vi "SetSheetColor.vi"() -> ()   [LabVIEW 2014]
panel:
  out "A0 2":string[][](table)
  in  "活动单元格:单元格背景色":u32(colorbox)
  in  "表格区域":cluster{"行":i32, " 列":i32, "大小":i32}
  in  "行":i32
  in  "列":i32
  in  "大小":i32
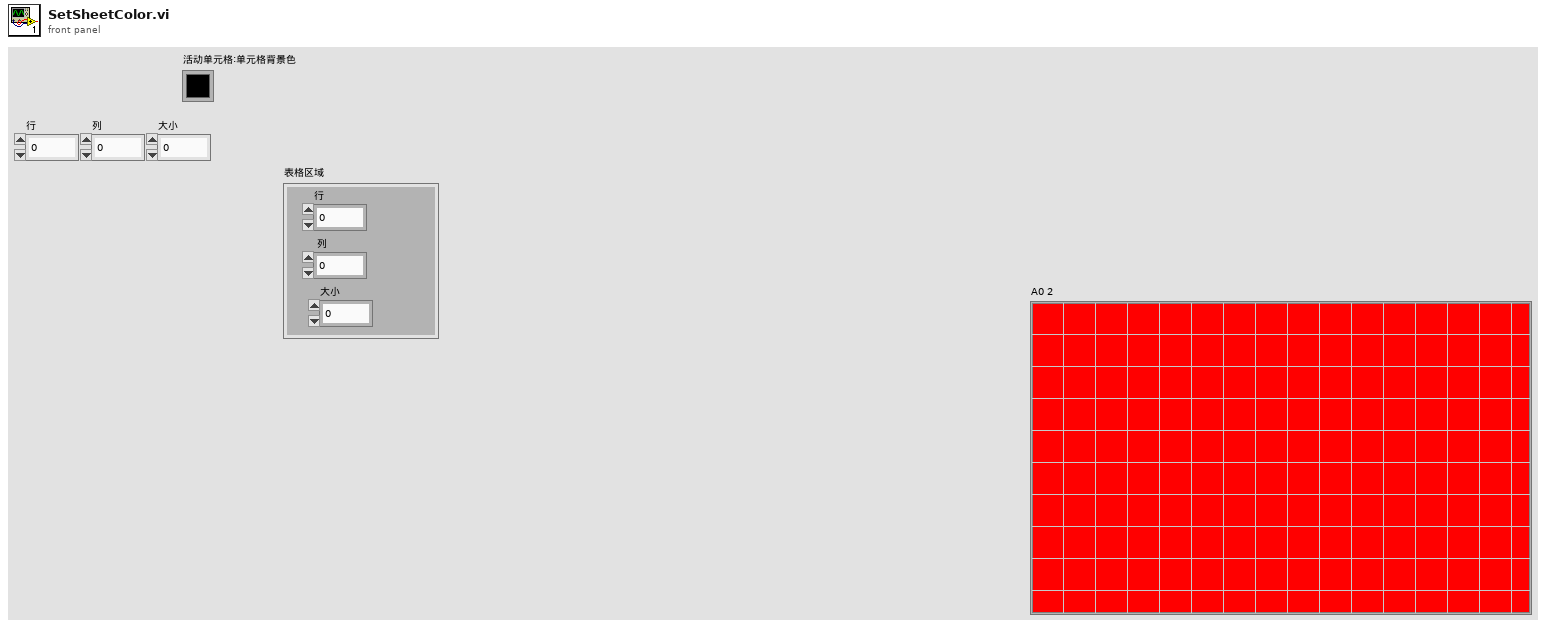
[diagram p1: front panel]
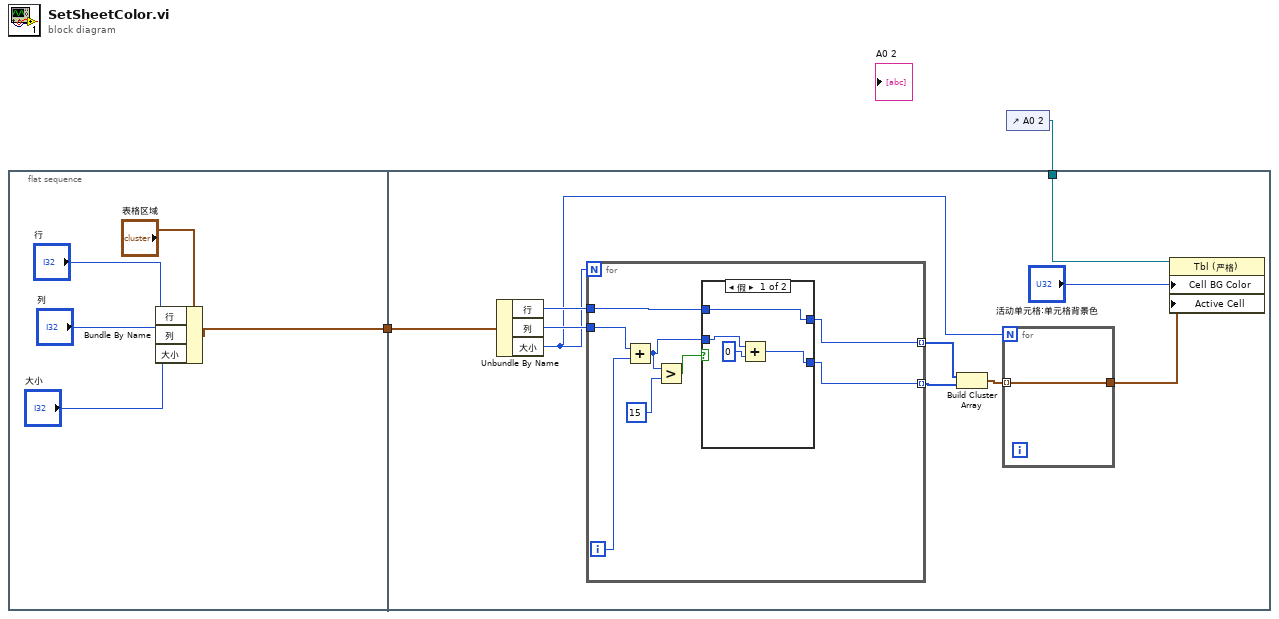
[diagram p0: block diagram]
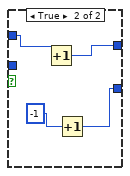
[diagram p2: hidden frame]
diagram:
  n1 = flat-sequence {
    tunnel: [w4] -> w2
    tunnel: w2 -> [w14]
    tunnel: w1 -> [w8]
    frame #0 {
      n2 = Bundle By Name(cluster="表格区域", "行"="行", "列"="列", "大小"="大小") -> (w4:cluster{"行":i32, " 列":i32, "大小":i32})
    }
    frame #1 {
      n3 = Unbundle By Name(w14) -> ("行"=w17:i32, "列"=w16:i32, "大小"=w11:i32)
      n4 = for {
        N: w11 -> [_]
        tunnel: w16 -> [w26]
        tunnel: w17 -> [w22]
        tunnel: [w20] -> w13 mode=indexing
        tunnel: [w19] -> w12 mode=indexing
        i -> [w23]
        n5 = Add(x=w26, y=w23) -> (x+y=w21:i32)
        n6 = Greater?(x=w21, y=u8 15) -> (0:w24:bool)
        n7 = case shown="假" w24 {
          tunnel: [w30 w34] -> w20
          tunnel: w22 -> [w30 w32]
          tunnel: [w27 w31] -> w19
          tunnel: w21 -> [w28 _]
          frame False {
            n8 = Add(x=w28, y=u8 0) -> (x+y=w27:i32)
          }
          frame True {
            n9 = Increment(x=w32) -> (x+1=w34:i32)
            n10 = Increment(x=-1) -> (x+1=w31:i32)
          }
        }
      }
      n11 = Build Cluster Array(w13, w12) -> (w10:cluster{"行":i32, i32}[])
      n12 = for {
        N: w11 -> [_]
        tunnel: w10 -> [w18] mode=indexing
        tunnel: [w18] -> w9
      }
      n13 = property on="属性节点" class="Tbl (严格)"(reference=w8, "Cell BG Color"="活动单元格:单元格背景色", "Active Cell"=w9) -> ()  [unwired: 1 in, 2 out]
    }
  }
  n14 = control-ref of="A0 2"() -> (w1:refnum<vi>)
